vi "Write MB session.vi"(8 "error in (no error)":errorcluster, 10 "MB Serial Master:MB_Master":refnum<class "MB_Master.lvclass">, 11 "Modicon PLC in":refnum<class "MB PLC Client.lvclass">) -> (0 "error out":errorcluster, 3 "Modicon PLC out":refnum<class "MB PLC Client.lvclass">)   [LabVIEW 2018, in "MB PLC Client.lvlib" / "MB PLC Client.lvclass"]
uses:
  MB PLC Client.lvclass
  <vilib>/Plasmionique/MB Master/MB_Master/MB_Master.lvclass
  MB PLC Client.lvclass/MB PLC Client.ctl
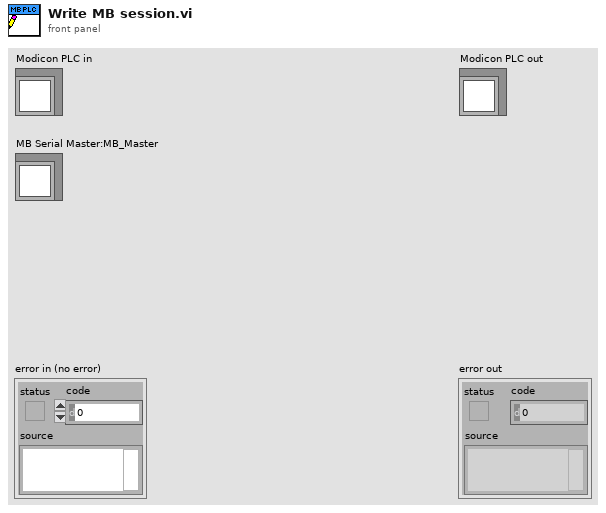
[diagram p1: front panel]
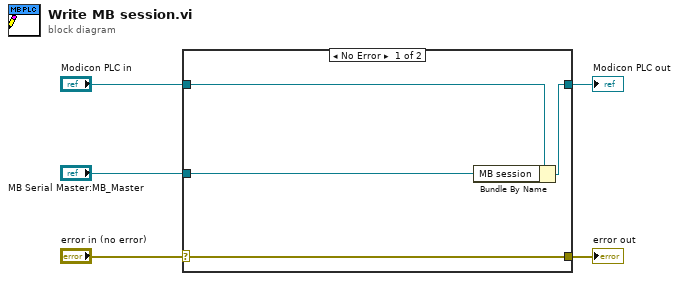
[diagram p0: block diagram]
diagram:
  n1 = case shown="No Error" "error in (no error)" {
    selector: "error in (no error)" -> [w9 w10]
    tunnel: [w9 w10] -> w4
    tunnel: [w7 w11] -> w2
    tunnel: "Modicon PLC in" -> [w8 w11]
    tunnel: "MB Serial Master:MB_Master" -> [w6 _]
    frame No Error {
      n2 = Bundle By Name(cluster=w8, "MB session"=w6) -> (w7:refnum<class "MB PLC Client.lvclass">)
    }
    frame Error {
    }
  }
  "error out" <- w4
  "Modicon PLC out" <- w2
